vi "_Check Server Lock.vi"(5 "LockServer":bool, 6 "Message In":string) -> (0 "error out":errorcluster, 2 "Message Out":string, 3 "Proceed":bool)   [LabVIEW 2015]
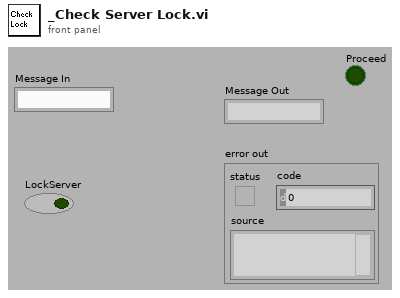
[diagram p1: front panel]
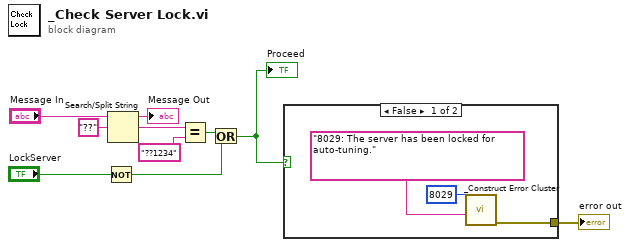
[diagram p0: block diagram]
diagram:
  n1 = Not(x="LockServer") -> (.not. x?=w10:bool)
  n2 = Search/Split String(string="Message In", search string/char (-)="??") -> (substring before match=→"Message Out":string, match + rest of string=w7:string)  [unwired: 2 out]
  n3 = Equal?(x=w7, y="??1234") -> (x = y?=w9:bool)
  n4 = Or(x=w9, y=w10) -> (x .or. y?=w2:bool)
  "Proceed" <- w2
  n5 = case shown="False" w2 {
    tunnel: [w11 _] -> w1
    frame False {
      n6 = call "_Construct Error Cluster.vi"("reason"="8029: The server has been locked for auto-tuning.", "errorCode"=8029) -> ("error out"=w11:errorcluster)  [unwired: 2 in, 3 out]
    }
    frame True {
    }
  }
  "error out" <- w1
